vi "Initialize Gyro.vi"   [LabVIEW 2018]
uses:
  gyro sensor adis/ADIS16448 IMU/ADIS16448_IMU.lvlib
types:
  T1 = typedef "ADIS16448_IMU.lvlib/ADI_IMU_ADIS16448_IMUDevRef.ctl" = cluster{"DevStatus":errorcluster, "Handle":i32, "SPI Bus":T2, "Device Found":bool, "Device Ready":bool, "Yaw Axis":enum16{"X", "Y", "Z"}, "AHRS Algorithm":enum16{"Complementary", "Madgwick"}, "Serial":u16, "Lot ID 2":u16, "Lot ID 1":u16, "Bytes Per Sample":u16, "Calibrate On Open?":bool}
  T2 = typedef "spi_bus.ctl" = enum16{"SPI On-Board, CS0", "SPI On-Board, CS1", "SPI On-Board, CS2", "SPI On-Board, CS3", "SPI MXP", "Invalid"}
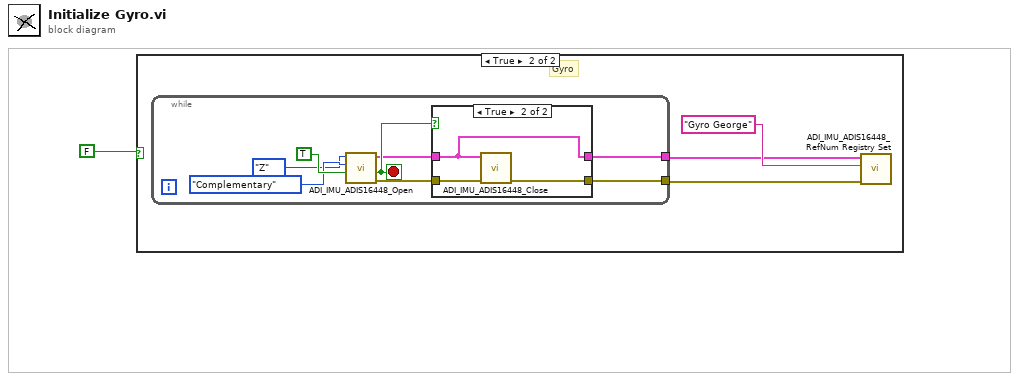
[diagram p0: block diagram]
diagram:
  n1 = case shown="True" FALSE {
    frame False {
    }
    frame True {
      # "Gyro"
      n2 = while {
        tunnel: [w5] -> w2
        tunnel: [w6] -> w3
        stop <- w9 stop-if-true
        n3 = call "ADI_IMU_ADIS16448_Open.vi"("Calibrate On Open 2"=TRUE ("Calibrate On Open"), "AHRS Algorithm 2"=enum16{"Complementary", "Madgwick"}."Complementary" ("AHRS Algorithm"), "Yaw Axis 2"=enum16{"X", "Y", "Z"}."Z" ("Yaw Axis")) -> ("error out 2"=w7:errorcluster, "error?"=w9:bool, "ADI IMU DevRef Out 2"=w8:T1)  [unwired: 6 in]
        n4 = case shown="True" w9 {
          tunnel: w8 -> [w14 w15]
          tunnel: w7 -> [w13 w17]
          tunnel: [w14 w15] -> w6
          tunnel: [w13 w16] -> w5
          frame False {
          }
          frame True {
            n5 = call "ADI_IMU_ADIS16448_Close.vi"("error in"=w17, "ADI IMU DevRef"=w15) -> ("error out"=w16:errorcluster)  [unwired: 9 in]
          }
        }
      }
      n6 = call "ADI_IMU_ADIS16448_RefNum Registry Set.vi"("error in (no error)"=w2, "refnum name"="Gyro George", "ADI IMU DevRef"=w3) -> ()  [unwired: 7 in, 2 out]
    }
  }
